vi "new RIO Device Filter.vi"(9 "RIO Device Name":string) -> (2 "RIO device filter out":refnum<class "Filter.lvclass">)   [LabVIEW 2016, in "RIO Device Filter.lvclass"]
uses:
  RIO Device Filter.lvclass
  Filter Parent/Filter.lvclass
  C:/github/VeriStand-FPGA-Resource-Manager/Source/Filters/Filter Parent/Filter.lvclass
  RIO Device Filter.lvclass/RIO Device Filter.ctl
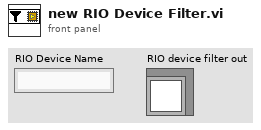
[diagram p1: front panel]
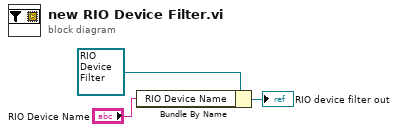
[diagram p0: block diagram]
diagram:
  n1 = Bundle By Name(cluster=refnum<class "RIO Device Filter.lvclass"> refnum ("RIO Device Filter in"), "RIO Device Name"="RIO Device Name") -> (→"RIO device filter out":refnum<class "RIO Device Filter.lvclass">)
